vi "UpdateStatus.vi"(8 "error in (no error)":errorcluster, 10 "status":string, 11 "Interface in":refnum<class "Interface.lvclass">) -> (0 "error out":errorcluster, 3 "Interface out":refnum<class "Interface.lvclass">)   [LabVIEW 2018, in "Interface.lvclass"]
uses:
  Interface.lvclass
  Interface.lvclass/Interface.ctl
panel:
  in  "Cluster CCD status":cluster{"CCD status":string}
  in  "Camera Status":T1
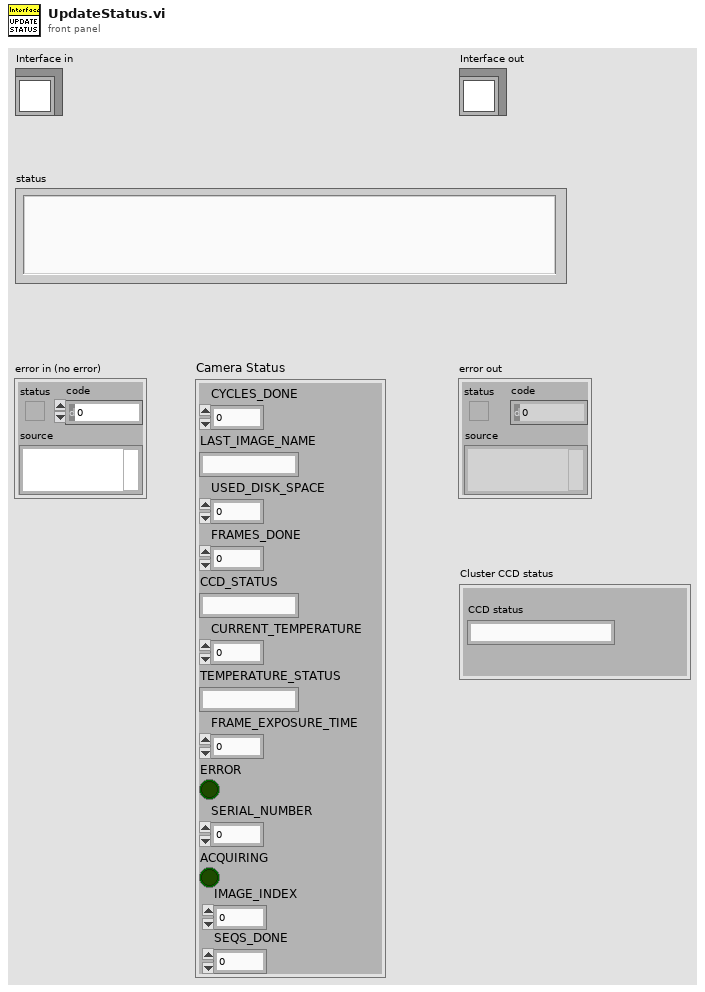
[diagram p1: front panel]
types:
  T1 = cluster{"CYCLES_DONE":u32, "LAST_IMAGE_NAME":string, "USED_DISK_SPACE":u16, "FRAMES_DONE":u16, "CCD_STATUS":string, "CURRENT_TEMPERATURE":i16, "TEMPERATURE_STATUS":string, "FRAME_EXPOSURE_TIME":dbl, "ERROR":bool, "SERIAL_NUMBER":u16, "ACQUIRING":bool, "SEQS_DONE":u32, "IMAGE_INDEX":u16}
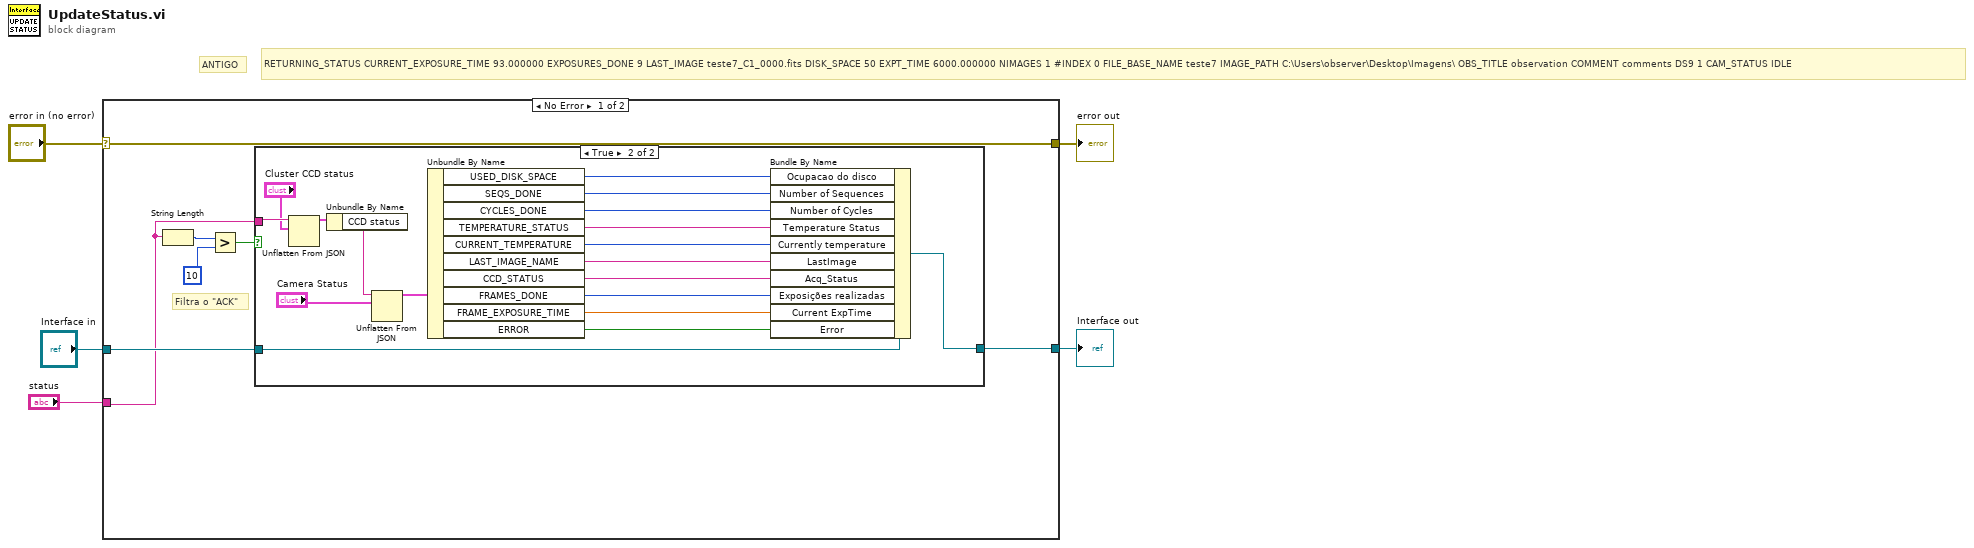
[diagram p0: block diagram]
diagram:
  # "ANTIGO"
  # "RETURNING_STATUS CURRENT_EXPOSURE_TIME 93.000000 EXPOSURES_DONE 9 LAST_IMAGE teste7_C1_0000.fits DISK_SPACE 50 EXPT_TIME 6000.000000 NIMAGES 1 #INDEX 0 FILE_BASE_NAME teste7 IMAGE_PATH C:\\Users\\observer\\Desktop\\Imagens\\ OBS_TITLE observation COMMENT comments DS9 1 CAM_STATUS IDLE"
  n1 = case shown="No Error" "error in (no error)" {
    selector: "error in (no error)" -> [w12 w33]
    tunnel: [w12 w33] -> w4
    tunnel: [w11 w32] -> w2
    tunnel: "Interface in" -> [w10 w32]
    tunnel: "status" -> [w9 _]
    frame No Error {
      # "Filtra o \"ACK\""
      n2 = String Length(string=w9) -> (length=w8:i32)
      n3 = Greater?(x=w8, y=10) -> (0:w6:bool)
      n4 = case shown="True" w6 {
        tunnel: [w13 w30] -> w11
        tunnel: w9 -> [_ w19]
        tunnel: w10 -> [w13 w31]
        frame False {
        }
        frame True {
          n5 = Unflatten From JSON(JSON string=w19, type and defaults="Cluster CCD status") -> (value=w17:cluster{"CCD status":string})  [unwired: 5 in, 1 out]
          n6 = Unbundle By Name(w17) -> ("CCD status"=w16:string)
          n7 = Unflatten From JSON(JSON string=w16, type and defaults="Camera Status") -> (value=w20:T1)  [unwired: 5 in, 1 out]
          n8 = Unbundle By Name(w20) -> ("USED_DISK_SPACE"=w15:u16, "SEQS_DONE"=w22:u32, "CYCLES_DONE"=w23:u32, "TEMPERATURE_STATUS"=w27:string, "CURRENT_TEMPERATURE"=w28:i16, "LAST_IMAGE_NAME"=w29:string, "CCD_STATUS"=w24:string, "FRAMES_DONE"=w26:u16, "FRAME_EXPOSURE_TIME"=w25:dbl, "ERROR"=w14:bool)
          n9 = Bundle By Name(cluster=w31, "Ocupacao do disco"=w15, "Number of Sequences"=w22, "Number of Cycles"=w23, "Temperature Status"=w27, "Currently temperature"=w28, "LastImage"=w29, "Acq_Status"=w24, "Exposições realizadas"=w26, "Current ExpTime"=w25, "Error"=w14) -> (w30:refnum<class "Interface.lvclass">)
        }
      }
    }
    frame Error {
    }
  }
  "error out" <- w4
  "Interface out" <- w2
